vi "MA3_Revolutions.vi"(1 "CW is Up":bool=TRUE, 2 "V in":dbl) -> (0 "Revs":dbl)   [LabVIEW 2015]
doc: "Help by FRC Team 836 - The RoboBees\n\nMA3 Revolutions\nThis VI monitors an absolute analog sensor output and reports position."
uses:
  <vilib>/Rock Robotics/SystemInterfaces/Typedef/FPGA_TypedefAnalogModule.ctl
  <vilib>/Rock Robotics/SystemInterfaces/AI/FPGA_AIChannel.ctl
panel:
  out "Rev s":dbl
  # "Example only"
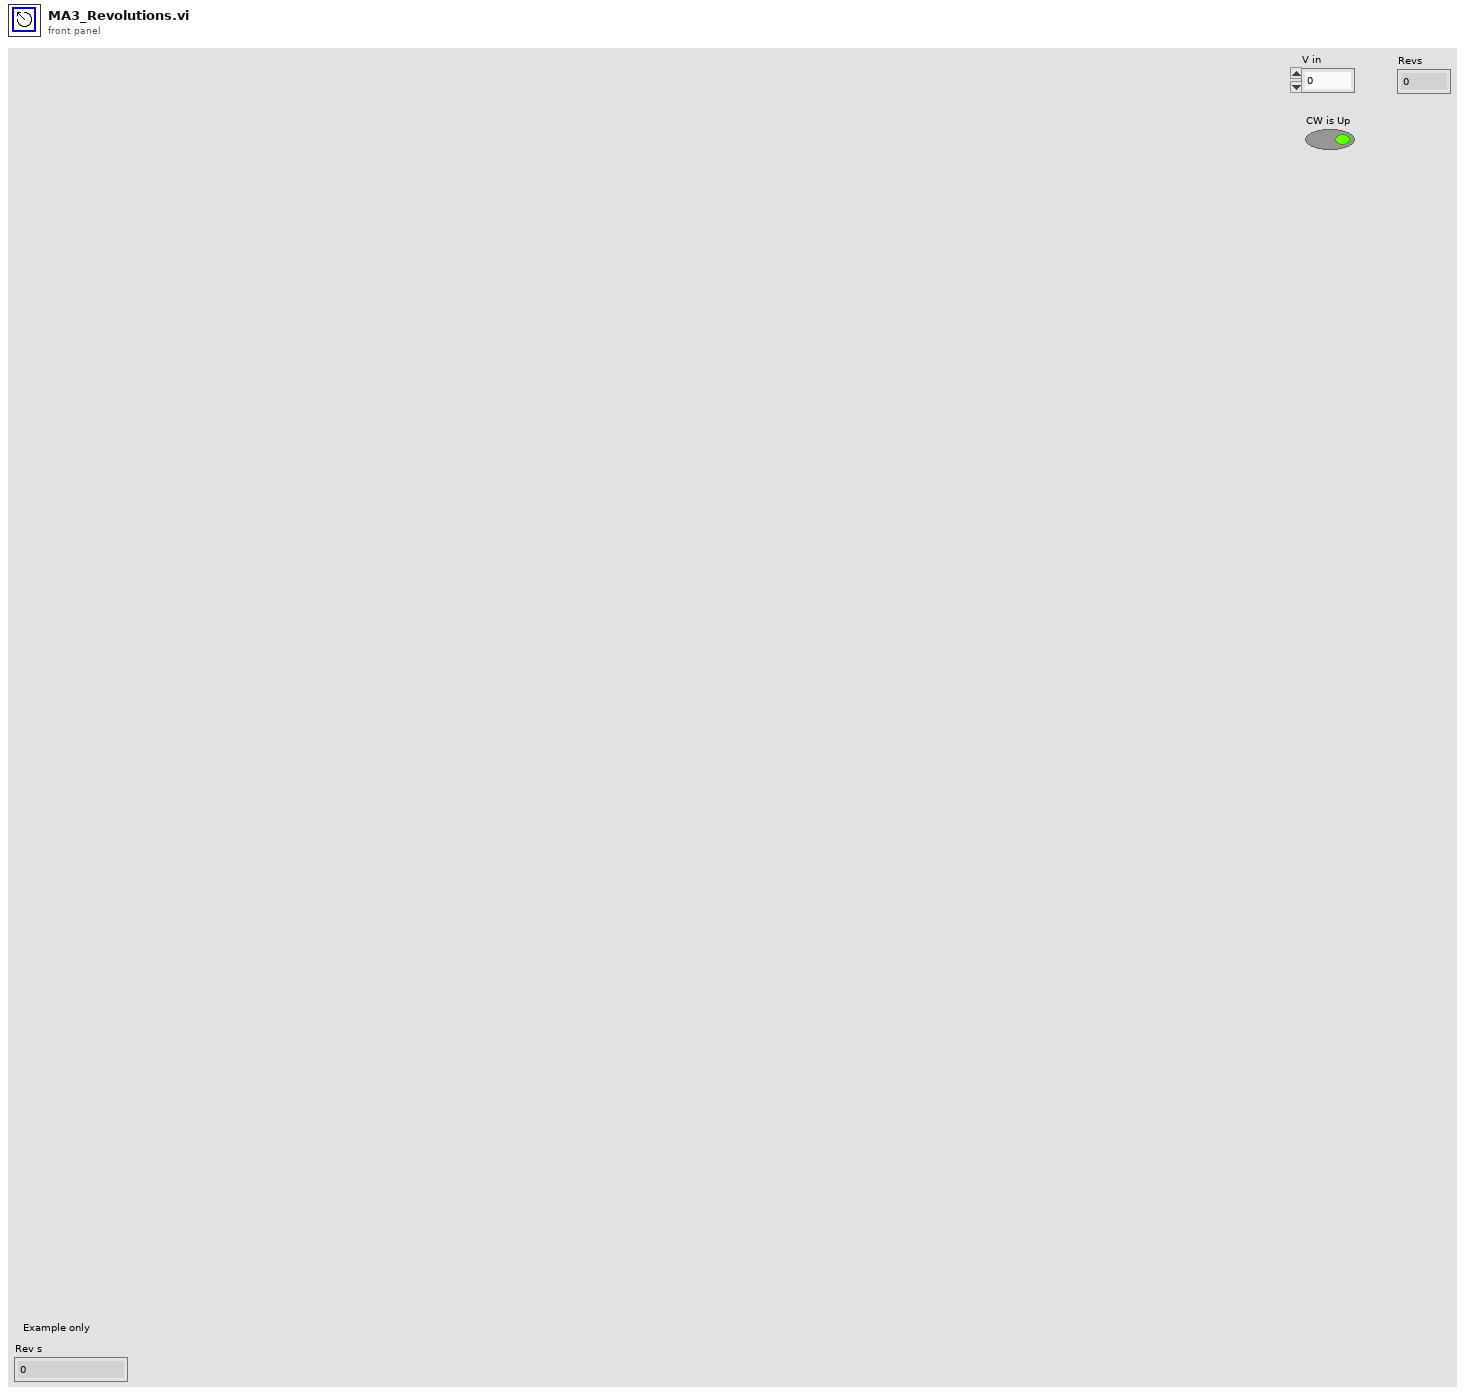
[diagram p1: front panel]
types:
  T1 = typedef "FPGA_AIChannel.ctl" = enum8{"AI 0", "AI 1", "AI 2", "AI 3", "AI MXP 0", "AI MXP 1", "AI MXP 2", "AI MXP 3", "Invalid"}
  T2 = typedef "FPGA_TypedefAnalogModule.ctl" = enum16{"Analog Module 1", "Analog Module 2"}
  T3 = typedef "WPI_AnalogChannelDevRef.ctl" = cluster{"DevStatus":errorcluster, "Analog Channel":T1}
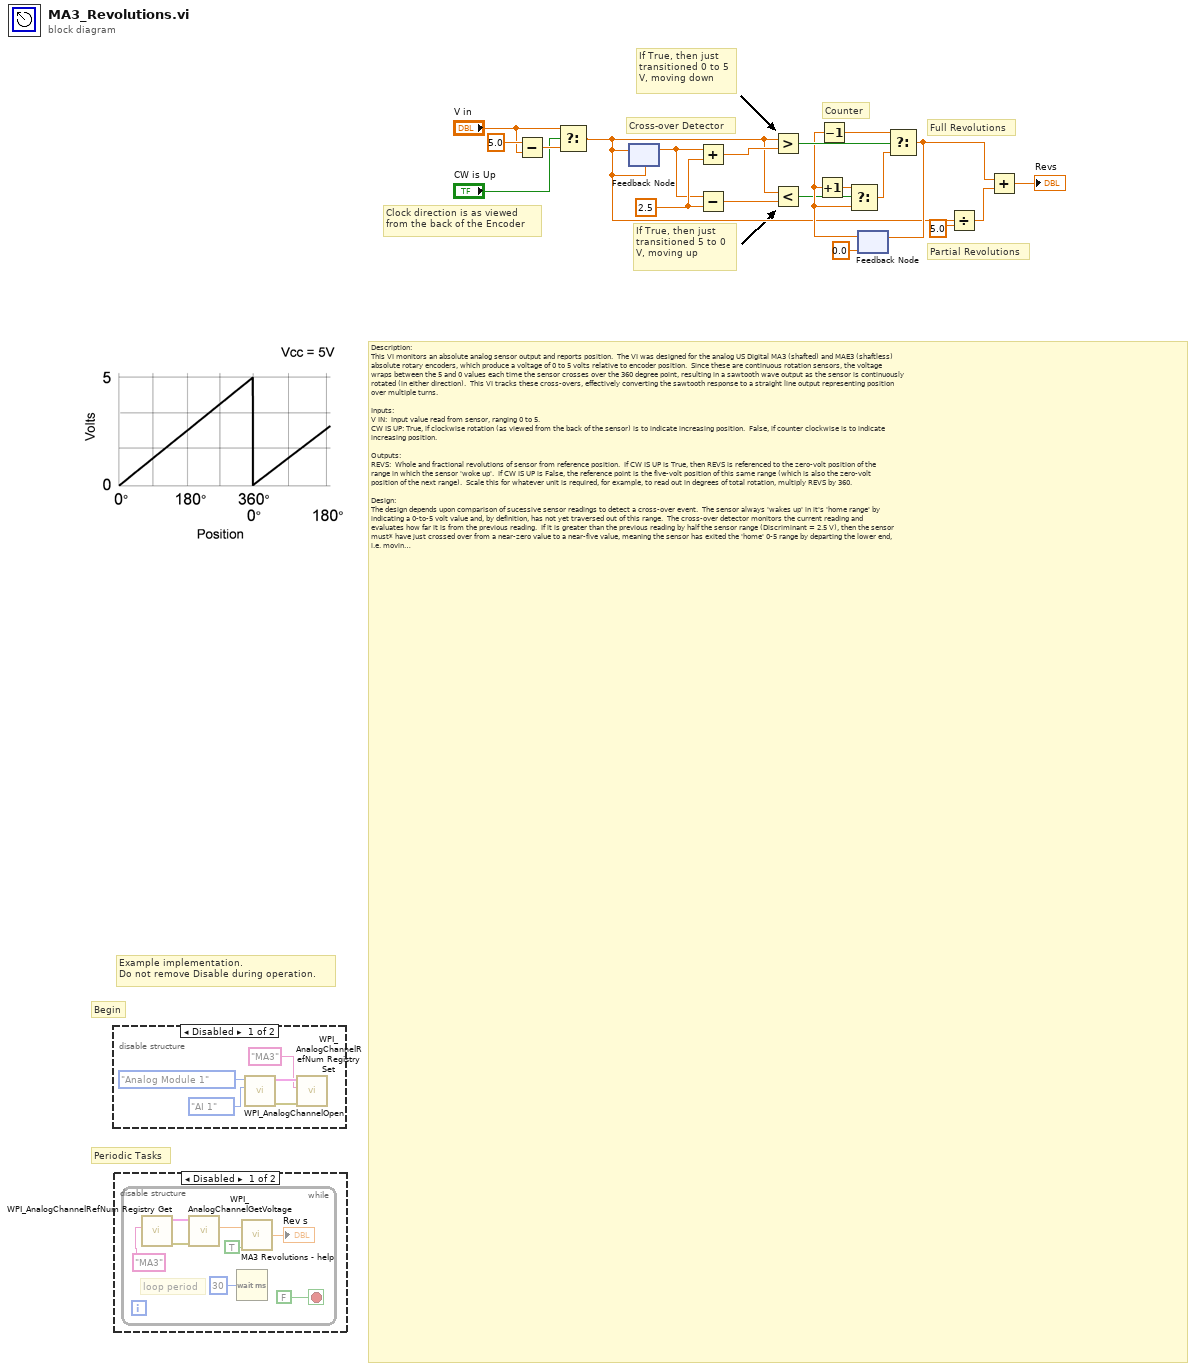
[diagram p0: block diagram]
diagram:
  w19 = 2.5 ("y")
  # "Begin"
  # "Periodic Tasks"
  # "Example implementation.\nDo not remove Disable during operation."
  # "Counter"
  # "Cross-over Detector"
  # "Partial Revolutions"
  # "Full Revolutions"
  # "Clock direction is as viewed\nfrom the back of the Encoder"
  # "If True, then just transitioned 5 to 0 V, moving up"
  # "If True, then just transitioned 0 to 5 V, moving down"
  # "Description:\nThis VI monitors an absolute analog sensor output and reports position.  The VI was designed for the analog US Digital MA3 (shafted) and MAE3 (shaftless)\nabsolute rotary encoders, which produce a voltage of 0 to 5 volts relative to encoder position.  Since these are continuous rotation sensors, the voltage\nwraps between the 5 and 0 values each time the sensor crosses over the 360 degree point, resulting in a sawtooth wave output as the sensor is continuously\nrotated (in either direction).  This VI tracks these cross-overs, effectively converting the sawtooth response to a straight line output representing position \nover multiple turns.\n\nInputs:\nV IN:  Input value read from sensor, ranging 0 to 5.\nCW IS UP: True, if clockwise rotation (as viewed from the back of the sensor) is to indicate increasing position.  False, if counter clockwise is to indicate\nincreasing position.\n\nOutputs:\nREVS:  Whole and fractional revolutions of sensor from reference position.  If CW IS UP is True, then REVS is referenced to the zero-volt position of the \nrange in which the sensor 'woke up'.  If CW IS UP is False, the reference point is the five-volt position of this same range (which is also the zero-volt \nposition of the next range).  Scale this for whatever unit is required, for example, to read out in degrees of total rotation, multiply REVS by 360.\n\nDesign:\nThe design depends upon comparison of sucessive sensor readings to detect a cross-over event.  The sensor always 'wakes up' in it's 'home range' by\nindicating a 0-to-5 volt value and, by definition, has not yet traversed out of this range.  The cross-over detector monitors the current reading and \nevaluates how far it is from the previous reading.  If it is greater than the previous reading by half the sensor range (Discriminant = 2.5 V), then the sensor \nmust* have just crossed over from a near-zero value to a near-five value, meaning the sensor has exited the 'home' 0-5 range by departing the lower end, \ni.e. moving down.  Similarly, if the current reading is less than the previous reading by half the sensor range, then the sensor must* have just crossed \nover from a near-five value to a near-zero value, meaning the sensor has exited the 'home' 0-5 range by departing the upper end, i.e. moving up.  The \nVI maintains a count of the range cross-overs to track the number and direction of ranges traversed - which are full revolutions of the sensor.  This is \nadded to the current fractional reading to indicate a complete absolute position from the home-zero ... even for multiple arbitrary range cross-overs.\n\nFor the MA(E)3 sensors, 2.5 is the optimum value for the discriminate (true for any 0-to-5 V range device) for best tolerance to noise and sampling rate.\nThe subVI can be easily altered for other range sizes (say, 0 to 10 V) - just be sure to also adjust the discriminant to the halfway point in the range. \n\n*The cross-over detector CAN be spoofed (falsely detect) under two circumstances.  Sucessive readings could be unintentionally seperated by the\ndiscriminate even if a cross-over has not occurred.  This can happen if (a) there is excessive sensor noise or (b) the loop cycle time is too slow for the \nsensor rate of change.   BOTH will contribute to the magnitude of sucessive reading difference ... a peak noise level of 0.5 Volt can by itself result in a 1.0 \nVolt excursion (peak-to-peak) over sucessive readings, worst case, under otherwise static conditions.  The cycle time for the loop where the sensor read is \nlocated effectively limits the sampling rate while the sensor value is changing - slow sampling of a relatively fast moving reading can also produce a large \ndifference in sucessive readings, which can fool the cross-over detector into counting this as a cross-over - when it isn't.\n\nTo prevent the possibility of these cross-over false detects, the sampling rate / loop cycle time must be sufficiently fast given the amount of peak noise \npresent and the maximum rate at which the sensor might rotate.   The principle is that the peak-to-peak noise plus the product of the max sensor rate of \nchange and the loop period must be less than the discriminant.  Solving for the loop period ...\n\n                                                           Loop Period < (2.5 - 2*n) / (5 * Sensor RPS)\nwhere:\n                                                           n = peak noise level, in volts\n                                                           Sensor RPS = maximum rate the sensor might change, in revolutions per second\n                                                           Loop Period = minimum required sampling rate of sensor, in seconds\n\nFor example, with a peak noise level of 0.25 Volts and a mechanical design requiring the sensor to rotate at 8 revolutions per second, the loop period \nmust be no slower than 50 milli-seconds to guarentee the subVI will reliably report how far the sensor has rotated.  The MA3 Sleeve Bushing model is \nspec'd as 100 RPM max shaft speed, or only ~1.7 revs per second, so the example is not practical for this MA3 but may be for another device.  (The \nBall Bearing version of the MA3 is spec'd at 15,000 RPM, or ~250 revs per sec).   A loop period safety margin may be warrented if the sensor read loop \nis prone to non-deterministic delays, otherwise, a timed loop could be used to ensure determinism (meaning the loop always executes on time) - IOW,\ndon't use the minimum required loop period for the sensor read unless you're confident that the loop will ALWAYS run that fast. \n\nImplementation:\nThis subVI is not needed if only using the sensor over a portion of one range.  If this is the case, just read the sensor directly.\nIf the MA(E)3 (or any sensor that continuously rotates and wraps 5 to 0 volts) is to be used across multiple ranges - note the sensor noise level in volts\nand how fast the sensor might rotate in revs per second, then use the Loop Period relation above to determine the minimum required Loop Period and\nensure the sensor is continuously read at this period or faster.\nCode using example at left.  Connect mechanism and run it through entire operating range.  Determine if clockwise or counter clockwise sensor rotation\nis to represent increasing position and set CW IS UP (T/F) as appropriate.  Determine if output needs to be scaled in rotational or linear displacement units \n(i.e. degrees or inches, for example).  Now the sensor will always report a consistent, unique, absolute position of the mechinism over its entire range, \ndespite power interruptions, AS LONG AS the mechanism wakes (powers) up in a consistent range.  This means that you must be careful to always put the\nphysical mechinism in the same general position before the system is powered up - this starting position does not need to be exact, just somewhere within\none 0-to-5 V sensor range that always corresponds with a particular mechanism position.\n\n\n----- RoboBees Team 836! -----  The more you DO, the more you CAN do.  If you like problem solving, think about a career in STEM! ..."
  n1 = disable-structure shown="Disabled" {
    frame Disabled {
      n2 = call <vilib>:"WPI_AnalogChannelOpen.vi"("Analog Channel"=FPGA_AIChannel."AI 1", 11:FPGA_TypedefAnalogModule."Analog Module 1" ("Analog Module (Module 1)")) -> ("error out"=w25:errorcluster, "AIDeviceRef"=w24:T3)  [unwired: 8 in]
      n3 = call <vilib>:"WPI_AnalogChannelRefNum Registry Set.vi"("error in (no error)"=w25, "refnum name"="MA3", "AIDeviceRef"=w24) -> ()  [unwired: 7 in, 2 out]
    }
    frame Enabled {
    }
  }
  n4 = disable-structure shown="Disabled" {
    frame Disabled {
      n5 = while {
        stop <- FALSE stop-if-true
        # "loop period"
        n6 = call <vilib>:"WPI_AnalogChannelRefNum Registry Get.vi"("refnum name"="MA3") -> ("error out"=w32:errorcluster, "AIDeviceRef"=w31:T3)  [unwired: 9 in]
        n7 = call <vilib>:"WPI_AnalogChannelGetVoltage.vi"("error in (no error)"=w32, "AIDeviceRef"=w31) -> ("Voltage"=w30:dbl)  [unwired: 7 in, 2 out]
        n8 = Wait (ms)(milliseconds to wait=u32 30) -> ()  [unwired: 1 out]
        n9 = call "MA3 Revolutions - help.vi"("CW is Up"=TRUE, "V in"=w30) -> ("Revs"=→"Rev s":dbl)
      }
    }
    frame Enabled {
    }
  }
  n10 = Subtract(x=5.0, y="V in") -> (x-y=w5:dbl)
  n11 = Select(t="V in", s="CW is Up", f=w5) -> (s? t:f=w4:dbl)
  n12 = feedback #1(w4) -> (w17:dbl)
  n13 = feedback-in #1(w4) -> ()
  n14 = Add(x=w17, y=w19) -> (x+y=w20:dbl)
  n15 = Subtract(x=w17, y=w19) -> (x-y=w18:dbl)
  n16 = Greater?(x=w4, y=w20) -> (0:w13:bool)
  n17 = Less?(x=w4, y=w18) -> (x < y?=w7:bool)
  n18 = feedback #2(0.0) -> (w9:dbl)
  n19 = Increment(x=w9) -> (x+1=w11:dbl)
  n20 = Decrement(x=w9) -> (x-1=w12:dbl)
  n21 = Select(t=w11, s=w7, f=w9) -> (s? t:f=w16:dbl)
  n22 = Select(t=w12, s=w13, f=w16) -> (s? t:f=w8:dbl)
  n23 = feedback-in #2(w8) -> ()
  n24 = Divide(x=w4, y=5.0) -> (x/y=w10:dbl)
  n25 = Add(x=w8, y=w10) -> (x+y=→"Revs":dbl)
